vi "JKI_Python_Server Example.vi"() -> ()   [LabVIEW 2013]
uses:
  Server/Register for Events (Single PyObject).vi
  Server/Server.lvclass
  Call/Call.lvclass
panel:
  in  "Show LabVIEW.py in Explorer":bool
  in  "Open Python":bool
  in  "Exit":bool
  out "Client Connected":bool
  out "error out":errorcluster
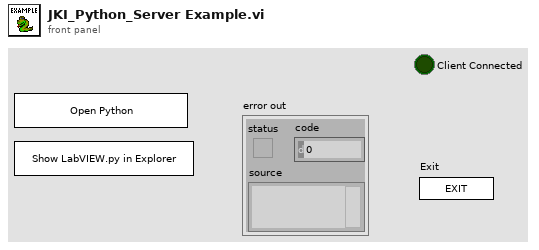
[diagram p1: front panel]
types:
  T1 = typedef "JKI_Python_Bridge_for_LV.lvlib/Server.lvclass/Python Method Call - Event Registration.ctl" = refnum<event-registration>
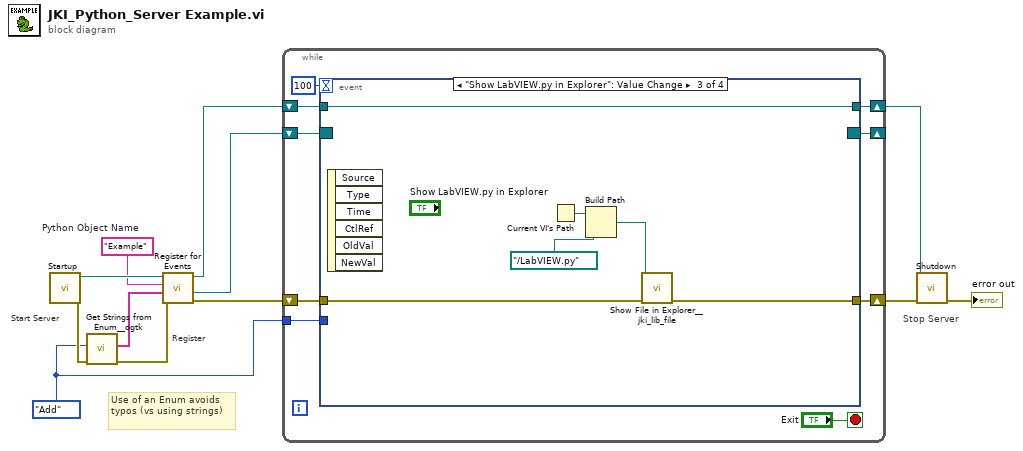
[diagram p0: block diagram]
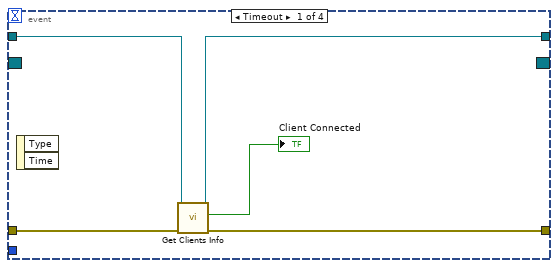
[diagram p2: hidden frame]
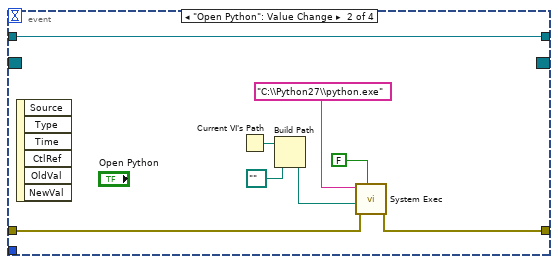
[diagram p3: hidden frame]
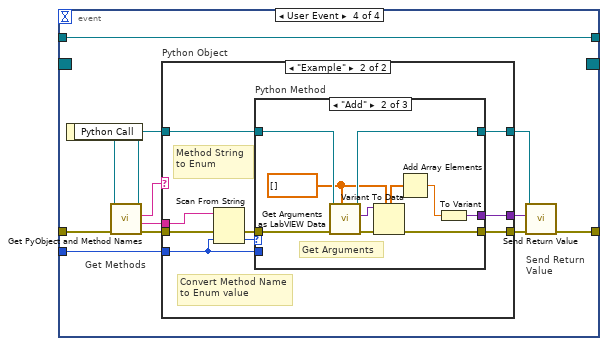
[diagram p4: hidden frame]
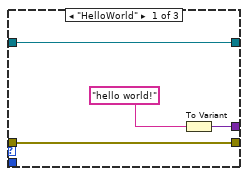
[diagram p6: hidden frame]
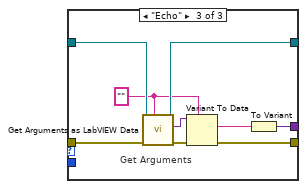
[diagram p7: hidden frame]
diagram:
  w4 = enum16{"HelloWorld", "Echo", "Add"}."Add"
  w1 = "Example"  # Python Object Name
  # "Use of an Enum avoids typos (vs using strings)"
  # "Register"
  # "Stop Server"
  # "Start Server"
  n1 = call "Startup.vi"() -> ("error out"=w5:errorcluster, "JKI_Python_Server out"=w10:refnum<class "Server.lvclass">)  [unwired: 10 in]
  n2 = call <userlib>:"Get Strings from Enum__ogtk.vi"("error in (no error)"=w5, "Enum"=w4) -> ("error out"=w6:errorcluster, "Enum Strings"=w2:string[])  [unwired: 6 in, 2 out]
  n3 = call-poly "Register for Events.vi"("error in (no error)"=w6, "Method Names"=w2, "PyObject Name"=w1, "JKI_Python_Server in"=w10) -> ("error out"=w8:errorcluster, "Python"=w3:T1, "JKI_Python_Server out"=w9:refnum<class "Server.lvclass">)  [unwired: 5 in]
  n4 = while {
    shift-right: [w18] -> w7
    shift-left: w8 -> [w20]
    shift-right: [w16] -> w11
    shift-left: w9 -> [w17]
    shift-right: [w15] -> _
    shift-left: w3 -> [w21]
    tunnel: w4 -> [w13]
    stop <- "Exit" stop-if-true
    n5 = event shown="[2] \"Show LabVIEW.py in Explorer\": Value Change" {
      selector: w21 -> [_ _ _ _]
      dyn-events: [_ _ _ _] -> w15
      timeout: 100 -> [_ _ _ _]
      tunnel: [w24 w28 w36 w45] -> w18
      tunnel: w20 -> [w25 w29 w37 w50]
      tunnel: w17 -> [w26 w34 w40 w52]
      tunnel: [w22 w34 w40 w52] -> w16
      tunnel: w13 -> [_ _ _ w47]
      event Timeout {
        n6 = event-data() -> ()  [unwired: 1 in, 2 out]
        n7 = call "Get Clients Info.vi"("error in (no error)"=w25, "JKI_Python_Server in"=w26) -> ("error out"=w24:errorcluster, "Client Connected"=→"Client Connected":bool, "JKI_Python_Server out"=w22:refnum<class "Server.lvclass">)  [unwired: 5 in, 2 out]
      }
      event "Open Python": Value Change {
        n8 = event-data() -> ()  [unwired: 1 in, 6 out]
        n9 = Current VI's Path() -> (path=w33:path)
        n10 = Build Path(base path=w33, name or relative path=path "..") -> (appended path=w30:path)
        n11 = call <vilib>:"System Exec.vi"("wait until completion? (T)"=FALSE, "error in (no error)"=w29, "working directory"=w30, "command line"="C:\\Python27\\python.exe") -> ("error out"=w28:errorcluster)  [unwired: 4 in, 3 out]
      }
      event "Show LabVIEW.py in Explorer": Value Change {
        n12 = event-data() -> ()  [unwired: 1 in, 6 out]
        n13 = Current VI's Path() -> (path=w39:path)
        n14 = Build Path(base path=w39, name or relative path=path "../LabVIEW.py") -> (appended path=w35:path)
        n15 = call <vilib>:"Show File in Explorer__jki_lib_file.vi"("error in (no error)"=w37, "File to Show"=w35) -> ("error out"=w36:errorcluster)  [unwired: 9 in]
      }
      event User Event {
        # "Send Return\nValue"
        # "Get Methods"
        n16 = event-data() -> ("Python Call"=w51:refnum<class "Call.lvclass">)  [unwired: 1 in]
        n17 = call "Get PyObject and Method Names.vi"("error in (no error)"=w50, "Call in"=w51) -> ("error out"=w49:errorcluster, "Method Name"=w42:string, "PyObject Name"=w41:string, "Call out"=w48:refnum<class "Call.lvclass">)  [unwired: 6 in]
        n18 = case "Python Object" shown="\"Example\"" w41 {
          tunnel: w49 -> [w53 w56]
          tunnel: w48 -> [w54 w62]
          tunnel: w47 -> [_ w61]
          tunnel: [w53 w60] -> w46
          tunnel: [w54 w59] -> w44
          tunnel: [_ w58] -> w43
          tunnel: w42 -> [_ w57]
          frame Default {
          }
          frame "Example" {
            # "Convert Method Name to Enum value"
            # "Method String to Enum"
            n19 = Scan From String(input string=w57, error in=w56, default 1=w61) -> (error out=w55:errorcluster, output 1=w63:enum16{"HelloWorld", "Echo", "Add"})  [unwired: 2 in, 2 out]
            n20 = case "Python Method" shown="\"Add\"" w63 {
              tunnel: [w64 w68 w78] -> w58
              tunnel: w55 -> [w66 w71 w82]
              tunnel: [w66 w76 w86] -> w60
              tunnel: [w65 w73 w84] -> w59
              tunnel: w62 -> [w65 w74 w85]
              tunnel: w61 -> [_ _ _]
              frame "HelloWorld" {
                n21 = To Variant(anything="hello world!" ("Arguments")) -> (Variant=w64:variant)
              }
              frame "Add" {
                w69 = dbl[] []
                # "Get Arguments"
                n22 = call "Get Arguments as LabVIEW Data.vi"("type"=w69, "error in (no error)"=w71, "Call in"=w74) -> ("error out"=w70:errorcluster, "LabVIEW Data"=w72:variant, "Call out"=w73:refnum<class "Call.lvclass">)  [unwired: 6 in]
                n23 = Variant To Data(error in=w70, type=w69, Variant=w72) -> (data=w77:dbl[], error out=w76:errorcluster)
                n24 = Add Array Elements(numeric array=w77) -> (sum=w75:dbl)
                n25 = To Variant(anything=w75) -> (Variant=w68:variant)
              }
              frame "Echo" {
                w80 = ""
                # "Get Arguments"
                n26 = call "Get Arguments as LabVIEW Data.vi"("type"=w80, "error in (no error)"=w82, "Call in"=w85) -> ("error out"=w81:errorcluster, "LabVIEW Data"=w83:variant, "Call out"=w84:refnum<class "Call.lvclass">)  [unwired: 6 in]
                n27 = Variant To Data(error in=w81, type=w80, Variant=w83) -> (data=w79:string, error out=w86:errorcluster)
                n28 = To Variant(anything=w79) -> (Variant=w78:variant)
              }
            }
          }
        }
        n29 = call "Send Return Value.vi"("error in (no error)"=w46, "Return Value"=w43, "Response in"=w44) -> ("error out"=w45:errorcluster)  [unwired: 8 in]
      }
    }
  }
  n30 = call "Shutdown.vi"("error in (no error)"=w7, "JKI_Python_Server in"=w11) -> ("error out"=→"error out":errorcluster)  [unwired: 9 in]
